vi "Fetch and Save as TDMS.vi"(0 "VISA resource name":refnum<visa-resource-name>, 1 "Segment Index (0)":i32 format="%.0g", 2 "TDMS Path":path, 5 "Measurement Source (1: Channel 1)":i32(ring)=1 items=["Channel 1"=1, "Channel 2"=2, "Channel 3"=3, "Channel 4"=4, "Function 1"=5, "Function 2"=6, "Function 3"=7, "Function 4"=8, "Memory 1"=9, "Memory 2"=10, "Memory 3"=11, "Memory 4"=12, "POD 1"=41, "POD 2"=42], 7 "Number of Samples (1000)":i32=10000 caption="Number of Samples (10000)", 9 "Maximum Time (10000ms)":u32=10000, 11 "error in (no error)":errorcluster, 12 "Offset (0)":i32, 13 "Waveform Format (0: Int8)":u16(ring) items=["Int8", "Int16", "Double"]) -> (4 "VISA resource name out":refnum<visa-resource-name>, 6 "Waveform Information":T1, 10 "Written Samples":i32, 15 "error out":errorcluster)   [LabVIEW 2013, in "Agilent 90000 Series.lvlib"]
doc: "Fetches scaled/unscaled data points from the instrument and save them into a TDMS file on the specified format."
uses:
  Agilent 90000 Series.lvlib
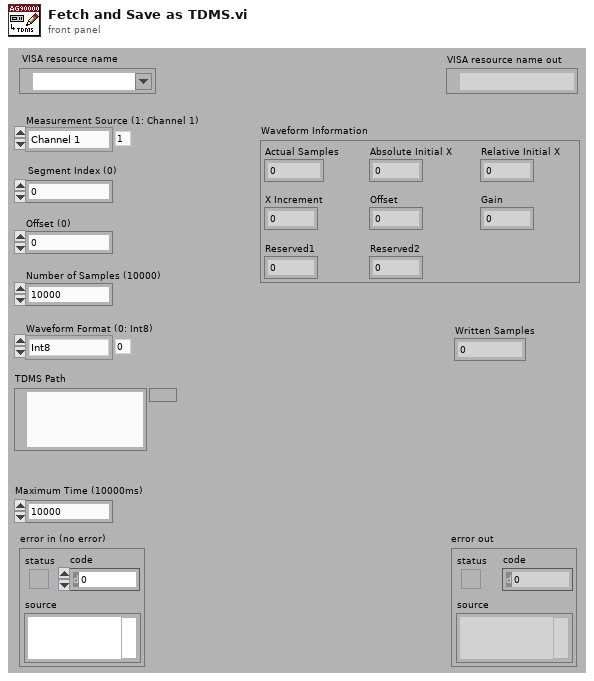
[diagram p1: front panel]
types:
  T1 = cluster{"Actual Samples":i32, "Absolute Initial X":dbl, "Relative Initial X":dbl, "X Increment":dbl, "Offset":dbl, "Gain":dbl, "Reserved1":dbl, "Reserved2":dbl}
  T2 = enum16{"open", "open or create", "create or replace", "create", "open (read-only)"}
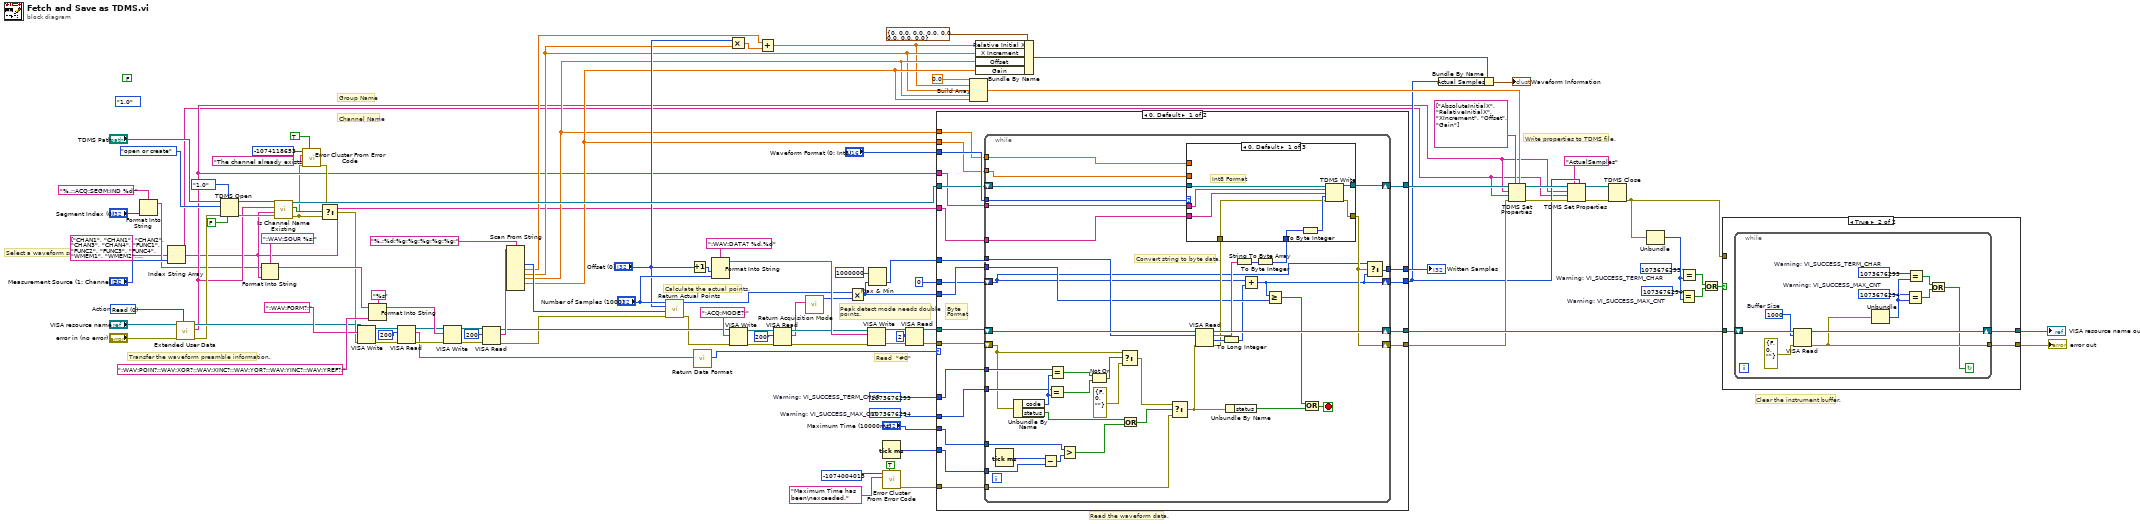
[diagram p0: block diagram]
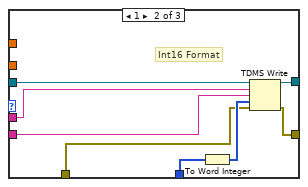
[diagram p2: hidden frame]
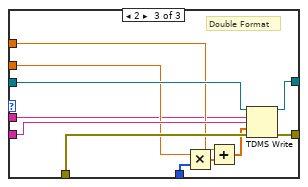
[diagram p3: hidden frame]
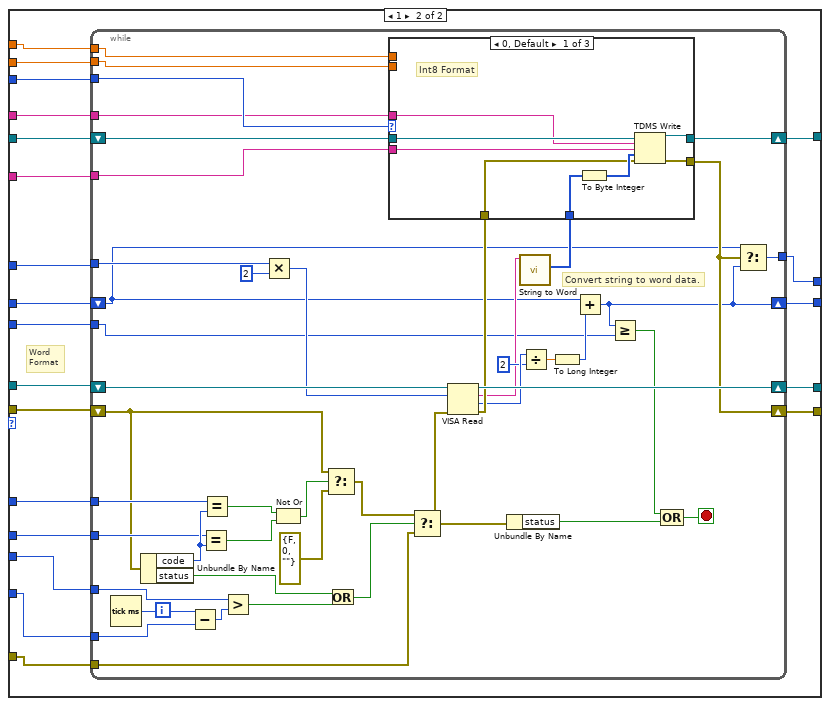
[diagram p4: hidden frame]
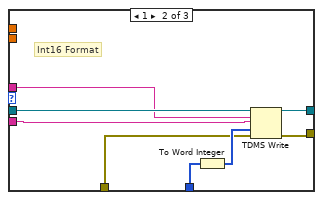
[diagram p5: hidden frame]
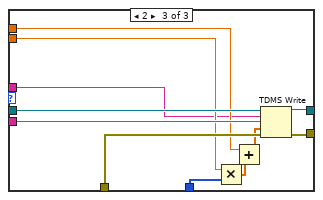
[diagram p6: hidden frame]
diagram:
  (unwired) FALSE ("disable buffering? (T)")
  (unwired) enum16{"1.0", "2.0"}."1.0" ("file format version (2.0)")
  (unwired) FALSE ("disable buffering? (T)")
  (unwired) enum16{"1.0", "2.0"}."1.0" ("file format version (2.0)")
  w17 = u16 0 items=["Read", "Write"]  # Action
  w86 = 1073676294  # Warning: VI_SUCCESS_MAX_CNT
  w87 = 1073676293  # Warning: VI_SUCCESS_TERM_CHAR
  w97 = 1073676294  # Warning: VI_SUCCESS_MAX_CNT
  w96 = 1073676293  # Warning: VI_SUCCESS_TERM_CHAR
  # "Group Name"
  # "Channel Name"
  # "Write properties to TDMS file."
  # "Peak detect mode needs double\npoints."
  # "Calculate the actual points."
  # "Read the waveform data."
  # "Read  \"#0\""
  # "Select a waveform source."
  # "Transfer the waveform preamble information."
  # "Clear the instrument buffer."
  n1 = Format Into String(format string="%.;:ACQ:SEGM:IND %d;", "Segment Index (0)") -> (resulting string=w5:string)  [unwired: 2 in, 1 out]
  n2 = Index String Array(1:"Measurement Source (1: Channel 1)", 2:string[] ["CHAN1", "CHAN1", "CHAN2", "CHAN3", "CHAN4", "FUNC1", "FUNC2", "FUNC3", "FUNC4", "WMEM1", "WMEM2", "WMEM3", "WMEM4", "AUX", "LINE", "CLOC", "MTR", "MSP", "EQU", "NONE", "DIG0", "DIG1", "DIG2", "DIG3", "DIG4", "DIG5", "DIG6", "DIG7", "DIG8", "DIG9", "DIG10", "DIG11", "DIG12", "DIG13", "DIG14", "DIG15", "", "", "", "", "", "POD1", "POD2", "", "", "", "", "", "", "", "", "BUS1", "BUS2", "BUS3", "BUS4", "", "", "", "", "", "", "DIFF1", "DIFF2", "", "", "", "", "", "", "", "", "COMM3", "COMM4"]) -> (0:w9:string)  [unwired: 1 out]
  n3 = call "Extended User Data.vi"("Action"=w17, "Error In (no error)"="error in (no error)", "VISA resource name in"="VISA resource name") -> ("Error Out"=w13:errorcluster, "Default Group Name Out"=w12:string, "VISA resource name out"=w15:refnum<visa-resource-name>)  [unwired: 1 in, 5 out]
  n4 = TDMS Open(6:FALSE ("disable buffering? (T)"), 7:enum16{"1.0", "2.0"}."1.0" ("file format version (2.0)"), 8:w13, 10:T2."open or create" ("operation (0:open)"), 11:"TDMS Path") -> (0:w70:errorcluster, 3:w69:refnum<k34>)  [unwired: 2 in]
  n5 = Format Into String(format string=":WAV:SOUR %s;" ("Source Command"), initial string=w5, w9) -> (resulting string=w106:string)  [unwired: 1 in, 1 out]
  n6 = call "Is Channel Name Existing.vi"("error in (no error)"=w70, "Channel Name"=w9, "Group Name"=w12, "TDMS File Ref In"=w69) -> ("error out"=w8:errorcluster, "Existed?"=w68:bool, "TDMS File Ref Out"=w67:refnum<k34>)  [unwired: 5 out]
  n7 = call <vilib>:"Error Cluster From Error Code.vi"("show call chain? (False)"=TRUE, "error in (no error)"=w8, "error message (\"\")"="The channel already exists." ("error message (\"\")"), "error code (0)"=-1074118653) -> ("error out"=w65:errorcluster)  [unwired: 5 out]
  n8 = Select(t=w65, s=w68, f=w8) -> (s? t:f=w38:errorcluster)
  n9 = VISA Write(VISA resource name=w15, write buffer=":WAV:FORM?;", error in (no error)=w38) -> (VISA resource name out=w61:refnum<visa-resource-name>, error out=w60:errorcluster)  [unwired: 1 out]
  n10 = Format Into String(format string="%s", initial string=w106, ":WAV:POIN?;:WAV:XOR?;:WAV:XINC?;:WAV:YOR?;:WAV:YINC?;:WAV:YREF?;" ("X/Y Increment, Origin, and Offset")) -> (resulting string=w105:string)  [unwired: 1 in, 1 out]
  n11 = VISA Read(VISA resource name=w61, byte count=u32 200, error in (no error)=w60) -> (VISA resource name out=w57:refnum<visa-resource-name>, read buffer=w55:string, error out=w56:errorcluster)  [unwired: 1 out]
  n12 = VISA Write(VISA resource name=w57, write buffer=w105, error in (no error)=w56) -> (VISA resource name out=w111:refnum<visa-resource-name>, error out=w110:errorcluster)  [unwired: 1 out]
  n13 = VISA Read(VISA resource name=w111, byte count=u32 200, error in (no error)=w110) -> (VISA resource name out=w50:refnum<visa-resource-name>, read buffer=w91:string, error out=w26:errorcluster)  [unwired: 1 out]
  n14 = Scan From String(format string="%.;%d;%g;%g;%g;%g;%g;", input string=w91) -> (output 1=w47:i32, output 2=w18:dbl, output 3=w20:dbl, output 4=w21:dbl, output 5=w22:dbl)  [unwired: 2 in, 10 out]
  n15 = call "Return Actual Points.vi"("error in (no error)"=w26, "Total Points (2000)"=w47, "Offset (0)"="Offset (0)", "Number of Samples (1000)"="Number of Samples (1000)") -> ("error out"=w25:errorcluster, "Actual Points"=w46:i32)  [unwired: 6 out]
  n16 = Increment(x="Offset (0)") -> (x+1=w23:i32)
  n17 = call "Return Data Format.vi"("String In"=w55) -> ("Data Format"=w11:u16)  [unwired: 10 out]
  n18 = Format Into String(format string=":WAV:DATA? %d,%d", w23, "Number of Samples (1000)") -> (resulting string=w89:string)  [unwired: 2 in, 1 out]
  n19 = Multiply(x="Offset (0)", y=w20) -> (x*y=w88:dbl)
  n20 = VISA Write(VISA resource name=w50, write buffer=":ACQ:MODE?;", error in (no error)=w25) -> (VISA resource name out=w53:refnum<visa-resource-name>, error out=w54:errorcluster)  [unwired: 1 out]
  n21 = Add(x=w18, y=w88) -> (x+y=w19:dbl)
  n22 = VISA Read(VISA resource name=w53, byte count=u32 200, error in (no error)=w54) -> (VISA resource name out=w49:refnum<visa-resource-name>, read buffer=w34:string, error out=w48:errorcluster)  [unwired: 1 out]
  n23 = call "Return Acquisition Mode.vi"("Acquisition Mode"=w34) -> ("Multiply Factor"=w35:i32)  [unwired: 10 out]
  n24 = Multiply(x=w46, y=w35) -> (x*y=w42:i32)
  n25 = VISA Write(VISA resource name=w49, write buffer=w89, error in (no error)=w48) -> (VISA resource name out=w94:refnum<visa-resource-name>, error out=w93:errorcluster)  [unwired: 1 out]
  n26 = Max & Min(x=1000000, y=w42) -> (min(x,y)=w74:i32)  [unwired: 1 out]
  n27 = Tick Count (ms)() -> (millisecond timer value=w84:u32)
  n28 = call <vilib>:"Error Cluster From Error Code.vi"("show call chain? (False)"=TRUE, "error message (\"\")"="Maximum Time has been\nexceeded." ("error message (\"\")"), "error code (0)"=-1074004013) -> ("error out"=w81:errorcluster)  [unwired: 1 in, 5 out]
  n29 = VISA Read(VISA resource name=w94, byte count=u32 2, error in (no error)=w93) -> (VISA resource name out=w62:refnum<visa-resource-name>, error out=w39:errorcluster)  [unwired: 2 out]
  n30 = case shown="0, Default" w11 {
    tunnel: [w132 w222] -> w102
    tunnel: [w131 w221] -> w72
    tunnel: w62 -> [w130 w220]
    tunnel: w87 -> [w129 w219]
    tunnel: w86 -> [w128 w218]
    tunnel: "Maximum Time (10000ms)" -> [w127 w217]
    tunnel: w84 -> [w113 w216]
    tunnel: w74 -> [w118 w206]
    tunnel: w81 -> [w126 w215]
    tunnel: w39 -> [w125 w214]
    tunnel: "Waveform Format (0: Int8)" -> [w124 w213]
    tunnel: w67 -> [w123 w212]
    tunnel: w9 -> [w122 w211]
    tunnel: w21 -> [w120 w209]
    tunnel: w22 -> [w121 w210]
    tunnel: [w114 w208] -> w71
    tunnel: w42 -> [w119 w207]
    tunnel: 0 ("index") -> [w117 w205]
    tunnel: [w116 w204] -> w36
    tunnel: [w115 w203] -> w28
    tunnel: w12 -> [w112 w202]
    frame 0, Default {
      # "Byte\nFormat"
      n31 = while {
        shift-right: [w138] -> w131
        shift-left: w125 -> [w163]
        shift-right: [w174] -> w132
        shift-left: w130 -> [w173]
        shift-right: [w136] -> w115
        shift-left: w117 -> [w137]
        tunnel: w129 -> [w165]
        tunnel: w128 -> [w164]
        tunnel: w127 -> [w160]
        tunnel: w113 -> [w159]
        tunnel: w126 -> [w154]
        tunnel: w124 -> [w149]
        shift-right: [w147] -> w114
        shift-left: w123 -> [w148]
        tunnel: w122 -> [w146]
        tunnel: w121 -> [w143]
        tunnel: w120 -> [w142]
        tunnel: w119 -> [w140]
        tunnel: w118 -> [w141]
        tunnel: [w135] -> w116
        tunnel: w112 -> [w133]
        stop <- w151 stop-if-true
        # "Convert string to byte data."
        n32 = Tick Count (ms)() -> (millisecond timer value=w161:u32)
        n33 = Unbundle By Name(w163) -> ("code"=w166:i32, "status"=w158:bool)
        n34 = Subtract(x=w161, y=w159) -> (x-y=w162:u32)
        n35 = Equal?(x=w164, y=w166) -> (x = y?=w169:bool)
        n36 = Equal?(x=w165, y=w166) -> (x = y?=w170:bool)
        n37 = Greater?(x=w160, y=w162) -> (0:w157:bool)
        n38 = Not Or(1:w169, 2:w170) -> (0:w168:bool)
        n39 = Select(t=w163, s=w168, f=errorcluster {"status"=FALSE, "code"=0, "source"=""} ("error in (no error)")) -> (s? t:f=w156:errorcluster)
        n40 = Or(x=w158, y=w157) -> (x .or. y?=w155:bool)
        n41 = Select(t=w156, s=w155, f=w154) -> (s? t:f=w153:errorcluster)
        n42 = VISA Read(VISA resource name=w173, byte count=w141, error in (no error)=w153) -> (VISA resource name out=w174:refnum<visa-resource-name>, read buffer=w150:string, return count=w172:u32, error out=w144:errorcluster)
        n43 = To Long Integer(number=w172) -> (32bit integer=w134:i32)
        n44 = Unbundle By Name(w153) -> ("status"=w152:bool)
        n45 = String To Byte Array(string=w150) -> (unsigned byte array=w145:u8[])
        n46 = Add(x=w137, y=w134) -> (x+y=w136:i32)
        n47 = To Byte Integer(number=w145) -> (8bit integer=w139:i8[])
        n48 = case shown="0, Default" w149 {
          tunnel: w148 -> [w182 w190 w201]
          tunnel: [w181 w189 w200] -> w147
          tunnel: w146 -> [w176 w184 w197]
          tunnel: w139 -> [w180 w188 w192]
          tunnel: w144 -> [w178 w186 w199]
          tunnel: [w177 w185 w198] -> w138
          tunnel: w143 -> [_ _ w193]
          tunnel: w142 -> [_ _ w194]
          tunnel: w133 -> [w175 w183 w191]
          frame 0, Default {
            # "Int8 Format"
            n49 = To Byte Integer(number=w180) -> (8bit integer=w179:i8[])
            n50 = TDMS Write(0:w182, 5:w175, 7:w176, 9:w179, 11:w178) -> (4:w181:refnum<k34>, 15:w177:errorcluster)  [unwired: 1 in, 2 out]
          }
          frame 1 {
            # "Int16 Format"
            n51 = To Word Integer(number=w188) -> (16bit integer=w187:i16[])
            n52 = TDMS Write(0:w190, 5:w183, 7:w184, 9:w187, 11:w186) -> (4:w189:refnum<k34>, 15:w185:errorcluster)  [unwired: 1 in, 2 out]
          }
          frame 2 {
            # "Double Format"
            n53 = Multiply(x=w193, y=w192) -> (x*y=w196:dbl[])
            n54 = Add(x=w194, y=w196) -> (x+y=w195:dbl[])
            n55 = TDMS Write(0:w201, 5:w191, 7:w197, 9:w195, 11:w199) -> (4:w200:refnum<k34>, 15:w198:errorcluster)  [unwired: 1 in, 2 out]
          }
        }
        n56 = Greater Or Equal?(x=w136, y=w140) -> (x >= y?=w171:bool)
        n57 = Compound Arithmetic op=OR(w171, w152) -> (w151:bool)
        n58 = Select(t=w137, s=w138, f=w136) -> (s? t:f=w135:i32)
      }
    }
    frame 1 {
      # "Word\nFormat"
      n59 = while {
        shift-right: [w229] -> w221
        shift-left: w214 -> [w257]
        shift-right: [w267] -> w222
        shift-left: w220 -> [w266]
        shift-right: [w226] -> w203
        shift-left: w205 -> [w227]
        tunnel: w219 -> [w259]
        tunnel: w218 -> [w258]
        tunnel: w217 -> [w223]
        tunnel: w216 -> [w254]
        tunnel: w215 -> [w249]
        tunnel: w213 -> [w245]
        shift-right: [w243] -> w208
        shift-left: w212 -> [w244]
        tunnel: w211 -> [w242]
        tunnel: w210 -> [w240]
        tunnel: w209 -> [w239]
        tunnel: w207 -> [w228]
        tunnel: w206 -> [w238]
        tunnel: [w225] -> w204
        tunnel: w202 -> [w224]
        stop <- w246 stop-if-true
        # "Convert string to word data."
        n60 = Tick Count (ms)() -> (millisecond timer value=w255:u32)
        n61 = Unbundle By Name(w257) -> ("code"=w260:i32, "status"=w253:bool)
        n62 = Subtract(x=w255, y=w254) -> (x-y=w256:u32)
        n63 = Equal?(x=w258, y=w260) -> (x = y?=w263:bool)
        n64 = Equal?(x=w259, y=w260) -> (x = y?=w264:bool)
        n65 = Greater?(x=w223, y=w256) -> (0:w252:bool)
        n66 = Multiply(x=w238, y=2) -> (x*y=w231:i32)
        n67 = Not Or(1:w263, 2:w264) -> (0:w262:bool)
        n68 = Select(t=w257, s=w262, f=errorcluster {"status"=FALSE, "code"=0, "source"=""} ("error in (no error)")) -> (s? t:f=w251:errorcluster)
        n69 = Or(x=w253, y=w252) -> (x .or. y?=w250:bool)
        n70 = Select(t=w251, s=w250, f=w249) -> (s? t:f=w248:errorcluster)
        n71 = VISA Read(VISA resource name=w266, byte count=w231, error in (no error)=w248) -> (VISA resource name out=w267:refnum<visa-resource-name>, read buffer=w232:string, return count=w236:u32, error out=w241:errorcluster)
        n72 = Unbundle By Name(w248) -> ("status"=w247:bool)
        n73 = call "String to Word.vi"("String"=w232) -> ("Int16 Data"=w233:i16[])  [unwired: 1 in, 9 out]
        n74 = case shown="0, Default" w245 {
          tunnel: w244 -> [w275 w283 w294]
          tunnel: [w274 w282 w293] -> w243
          tunnel: w242 -> [w269 w277 w290]
          tunnel: w233 -> [w273 w281 w285]
          tunnel: w241 -> [w271 w279 w292]
          tunnel: [w270 w278 w291] -> w229
          tunnel: w240 -> [_ _ w286]
          tunnel: w239 -> [_ _ w287]
          tunnel: w224 -> [w268 w276 w284]
          frame 0, Default {
            # "Int8 Format"
            n75 = To Byte Integer(number=w273) -> (8bit integer=w272:i8[])
            n76 = TDMS Write(0:w275, 5:w268, 7:w269, 9:w272, 11:w271) -> (4:w274:refnum<k34>, 15:w270:errorcluster)  [unwired: 1 in, 2 out]
          }
          frame 1 {
            # "Int16 Format"
            n77 = To Word Integer(number=w281) -> (16bit integer=w280:i16[])
            n78 = TDMS Write(0:w283, 5:w276, 7:w277, 9:w280, 11:w279) -> (4:w282:refnum<k34>, 15:w278:errorcluster)  [unwired: 1 in, 2 out]
          }
          frame 2 {
            n79 = Multiply(x=w286, y=w285) -> (x*y=w289:dbl[])
            n80 = Add(x=w287, y=w289) -> (x+y=w288:dbl[])
            n81 = TDMS Write(0:w294, 5:w284, 7:w290, 9:w288, 11:w292) -> (4:w293:refnum<k34>, 15:w291:errorcluster)  [unwired: 1 in, 2 out]
          }
        }
        n82 = Divide(x=w236, y=u32 2) -> (x/y=w237:dbl)
        n83 = To Long Integer(number=w237) -> (32bit integer=w234:i32)
        n84 = Add(x=w227, y=w234) -> (x+y=w226:i32)
        n85 = Greater Or Equal?(x=w226, y=w228) -> (x >= y?=w265:bool)
        n86 = Compound Arithmetic op=OR(w265, w247) -> (w246:bool)
        n87 = Select(t=w227, s=w229, f=w226) -> (s? t:f=w225:i32)
      }
    }
  }
  "Written Samples" <- w36
  n88 = Build Array(0.0 ("output 2"), w19, w20, w21, w22) -> (w77:dbl[])
  n89 = Bundle By Name(cluster=T1 {"Actual Samples"=0, "Absolute Initial X"=0.0, "Relative Initial X"=0.0, "X Increment"=0.0, "Offset"=0.0, "Gain"=0.0, "Reserved1"=0.0, "Reserved2"=0.0} ("Waveform Information"), "Relative Initial X"=w19, "X Increment"=w20, "Offset"=w21, "Gain"=w22) -> (w76:T1)
  n90 = Bundle By Name(cluster=w76, "Actual Samples"=w28) -> (→"Waveform Information":T1)
  n91 = TDMS Set Properties(5:w77, 7:string[] ["AbsoluteInitialX", "RelativeInitialX", "XIncrement", "Offset", "Gain"] ("property names"), 8:w72, 9:w9, 10:w12, 11:w71) -> (0:w32:errorcluster, 3:w29:refnum<k34>)  [unwired: 2 out]
  n92 = TDMS Set Properties(5:w28, 7:"ActualSamples" ("property names"), 8:w32, 9:w9, 10:w12, 11:w29) -> (0:w31:errorcluster, 3:w30:refnum<k34>)  [unwired: 2 out]
  n93 = TDMS Close(8:w31, 11:w30) -> (0:w10:errorcluster)  [unwired: 1 out]
  n94 = Unbundle(w10) -> ("code"=w98:i32)  [unwired: 2 out]
  n95 = Equal?(x=w97, y=w98) -> (x = y?=w100:bool)
  n96 = Equal?(x=w96, y=w98) -> (x = y?=w101:bool)
  n97 = Or(x=w101, y=w100) -> (x .or. y?=w99:bool)
  n98 = case shown="True" w99 {
    tunnel: w102 -> [w296 w299]
    tunnel: w10 -> [w295 _]
    tunnel: [w296 w298] -> w43
    tunnel: [w295 w297] -> w44
    frame False {
    }
    frame True {
      n99 = while {
        shift-right: [w309] -> w298
        shift-left: w299 -> [w310]
        tunnel: [w302] -> w297
        stop <- w301 continue-if-true
        w304 = 1073676294  # Warning: VI_SUCCESS_MAX_CNT
        w303 = 1073676293  # Warning: VI_SUCCESS_TERM_CHAR
        w308 = u32 1000  # Buffer Size
        n100 = VISA Read(VISA resource name=w310, byte count=w308, error in (no error)=errorcluster {"status"=FALSE, "code"=0, "source"=""}) -> (VISA resource name out=w309:refnum<visa-resource-name>, error out=w302:errorcluster)  [unwired: 2 out]
        n101 = Unbundle(w302) -> ("code"=w305:i32)  [unwired: 2 out]
        n102 = Equal?(x=w304, y=w305) -> (x = y?=w306:bool)
        n103 = Equal?(x=w303, y=w305) -> (x = y?=w307:bool)
        n104 = Or(x=w307, y=w306) -> (x .or. y?=w301:bool)
      }
    }
  }
  "error out" <- w44
  "VISA resource name out" <- w43
